vi "Disconnect.vi"(8 "error in (no error)":errorcluster, 11 "Process in":refnum<class "Process.lvclass">) -> (0 "error out":errorcluster, 3 "Process out":refnum<class "Process.lvclass">)   [LabVIEW 2017, in "Process.lvclass"]
uses:
  Process.lvclass
  Process.lvclass/Process.ctl
  DLL/Modbus.dll
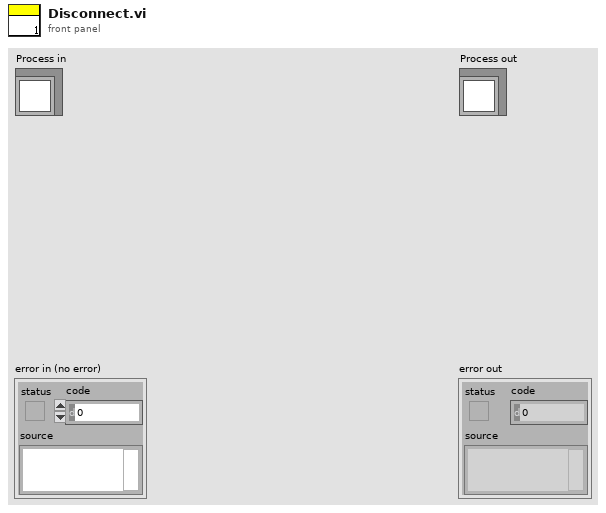
[diagram p1: front panel]
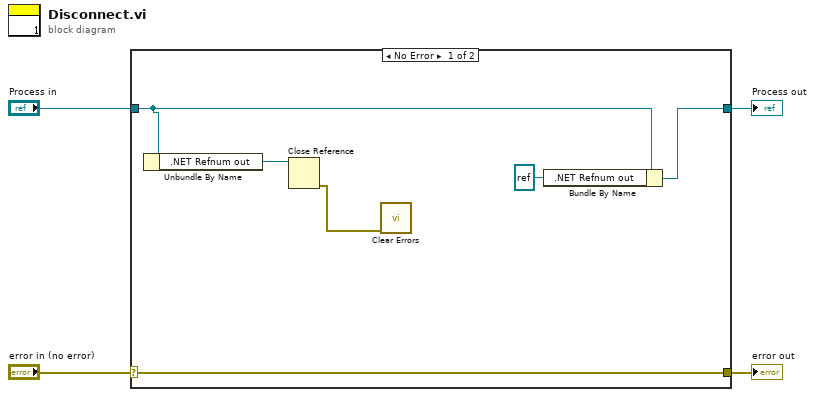
[diagram p0: block diagram]
diagram:
  n1 = case shown="No Error" "error in (no error)" {
    selector: "error in (no error)" -> [w10 w12]
    tunnel: [w10 w12] -> w3
    tunnel: [w8 w11] -> w1
    tunnel: "Process in" -> [w9 w11]
    frame No Error {
      n2 = Unbundle By Name(w9) -> (".NET Refnum out"=w7:refnum<k24>)
      n3 = Close Reference(reference=w7) -> (error out=w6:errorcluster)  [unwired: 1 in]
      n4 = call <vilib>:"Clear Errors.vi"("error in (no error)"=w6) -> ()  [unwired: 5 in, 2 out]
      n5 = Bundle By Name(cluster=w9, ".NET Refnum out"=refnum<k24> refnum) -> (w8:refnum<class "Process.lvclass">)
    }
    frame Error {
    }
  }
  "error out" <- w3
  "Process out" <- w1
